vi "load data.vi"(7 "Data loaded reference In":refnum<data-value>, 9 "File Structure":T1, 10 "Data Form":T2, 11 "File Array In":path[](array[path])) -> (5 "Data loaded reference Out":refnum<data-value>)   [LabVIEW 2023]
uses:
  control/Data Form.ctl
  control/file structure.ctl
  <vilib>/Utility/file.llb/Read Delimited Spreadsheet (string).vi
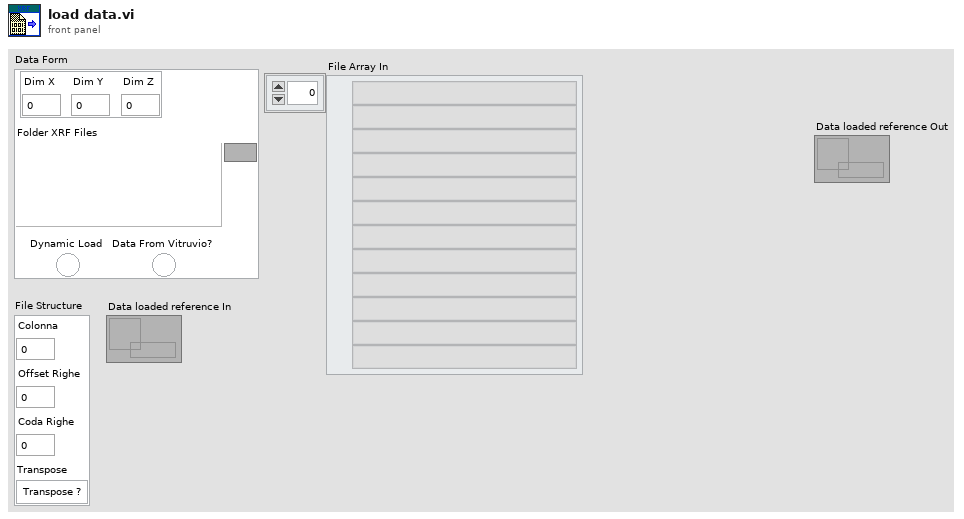
[diagram p1: front panel]
types:
  T1 = typedef "file structure.ctl" = cluster{"Colonna":i32, "Offset Righe":i32, "Coda Righe":i32, "Transpose":bool}
  T2 = typedef "Data Form.ctl" = cluster{"Dimensions":cluster{"Dim X":i32, "Dim Y":i32, "Dim Z":i32}, "Folder XRF Files":path, "Dynamic Load":bool, "Data From Vitruvio?":bool}
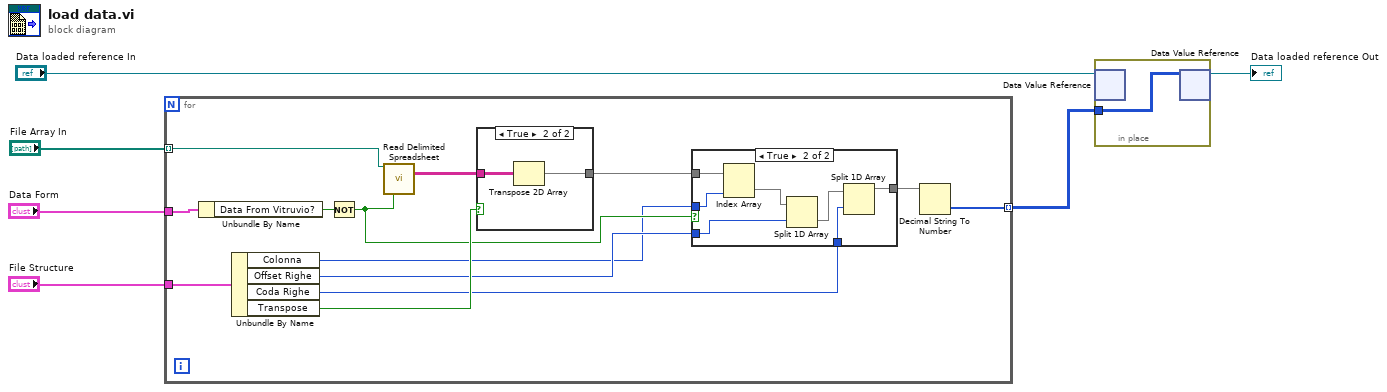
[diagram p0: block diagram]
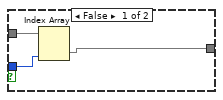
[diagram p2: hidden frame]
diagram:
  n1 = for {
    tunnel: "File Array In" -> [w17] mode=indexing
    tunnel: "Data Form" -> [w19]
    tunnel: "File Structure" -> [w16]
    tunnel: [w7] -> w3 mode=indexing
    n2 = Unbundle By Name(w19) -> ("Data From Vitruvio?"=w18:bool)
    n3 = Unbundle By Name(w16) -> ("Colonna"=w9:i32, "Offset Righe"=w14:i32, "Coda Righe"=w13:i32, "Transpose"=w15:bool)
    n4 = Not(x=w18) -> (.not. x?=w11:bool)
    n5 = call-poly <vilib>:"Read Delimited Spreadsheet.vi"("file path (dialog if empty)"=w17, "transpose? (F)"=w11) -> ("all rows"=w12:string[][])  [unwired: 8 in, 5 out]
    n6 = case shown="True" w15 {
      tunnel: w12 -> [w30 w32]
      tunnel: [w30 w31] -> w10
      frame False {
      }
      frame True {
        n7 = Transpose 2D Array(2D array=w32) -> (transposed array=w31:string[][])
      }
    }
    n8 = case shown="True" w11 {
      tunnel: w14 -> [_ w29]
      tunnel: w13 -> [_ w27]
      tunnel: [w21 w26] -> w8
      tunnel: w10 -> [w22 w25]
      tunnel: w9 -> [w20 w24]
      frame False {
        n9 = Index Array(array=w22, index (col)=w20) -> (element=w21:string[])  [unwired: 1 in]
      }
      frame True {
        n10 = Index Array(array=w25, index (col)=w24) -> (element=w23:string[])  [unwired: 1 in]
        n11 = Split 1D Array(array=w23, index=w29) -> (second subarray=w28:string[])  [unwired: 1 out]
        n12 = Split 1D Array(array=w28, index=w27) -> (first subarray=w26:string[])  [unwired: 1 out]
      }
    }
    n13 = Decimal String To Number(string=w8) -> (number=w7:i32[])  [unwired: 2 in, 1 out]
  }
  n14 = in-place {
    in-place-border: w3 -> [w33]
    n15 = in-place-dvr #1("Data loaded reference In") -> ()  [unwired: 2 out]
    n16 = in-place-dvr #1(w33) -> (→"Data loaded reference Out":refnum<data-value>)  [unwired: 1 out]
  }
